vi "Agilent 364xA (GPIB,Serial) Initialization VI.vi"(8 "error in (no error)":errorcluster, 10 "Custom XML":string, 11 "Device Item Ref in":T3 format="%.0x") -> (0 "error out":errorcluster, 3 "Device Item Ref out":T3 format="%.0x")   [LabVIEW 2009, in "Agilent 364xA (GPIB,Serial) Custom Device.lvlib"]
uses:
  Agilent 364xA (GPIB,Serial) Custom Device.lvlib
  <vilib>/NI VeriStand/Custom Device API/Custom Device Item Ref.ctl
  <vilib>/NI VeriStand/Custom Device API/Custom Device Channel.ctl
  <vilib>/NI VeriStand/Custom Device API/Custom Device Channel Type.ctl
  <vilib>/NI VeriStand/Custom Device API/Custom Device Loop Type.ctl
  <vilib>/NI VeriStand/Custom Device API/Custom Device API.lvlib
panel:
  in  "Enable Channel":T1={"Type"=enum."Input", "Units"="", "Default Value"=0.0, "Faultable"=TRUE, "Scalable"=FALSE}
  in  "Output Channels":T1={"Type"=enum."Output", "Units"="", "Default Value"=0.0, "Faultable"=FALSE, "Scalable"=FALSE}
  in  "Input Channels":T1={"Type"=enum."Input", "Units"="Amps", "Default Value"=0.0, "Faultable"=TRUE, "Scalable"=TRUE}
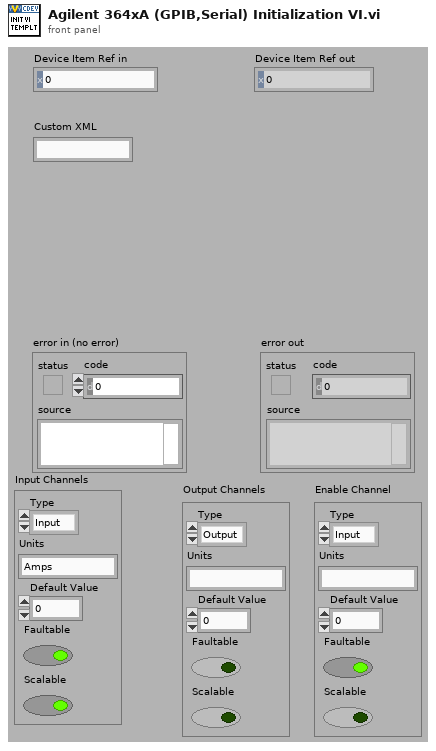
[diagram p1: front panel]
types:
  T1 = typedef "Custom Device API.lvlib/Custom Device Channel.ctl" = cluster{"Type":T2, "Units":string, "Default Value":dbl, "Faultable":bool, "Scalable":bool}
  T2 = typedef "Custom Device API.lvlib/Custom Device Channel Type.ctl" = enum16{"Input", "Output"}
  T3 = typedef "Custom Device API.lvlib/Custom Device Item Ref.ctl" = u64
  T4 = typedef "Custom Device API.lvlib/Custom Device Loop Type.ctl" = enum32{"While Loop", "Timed Loop"}
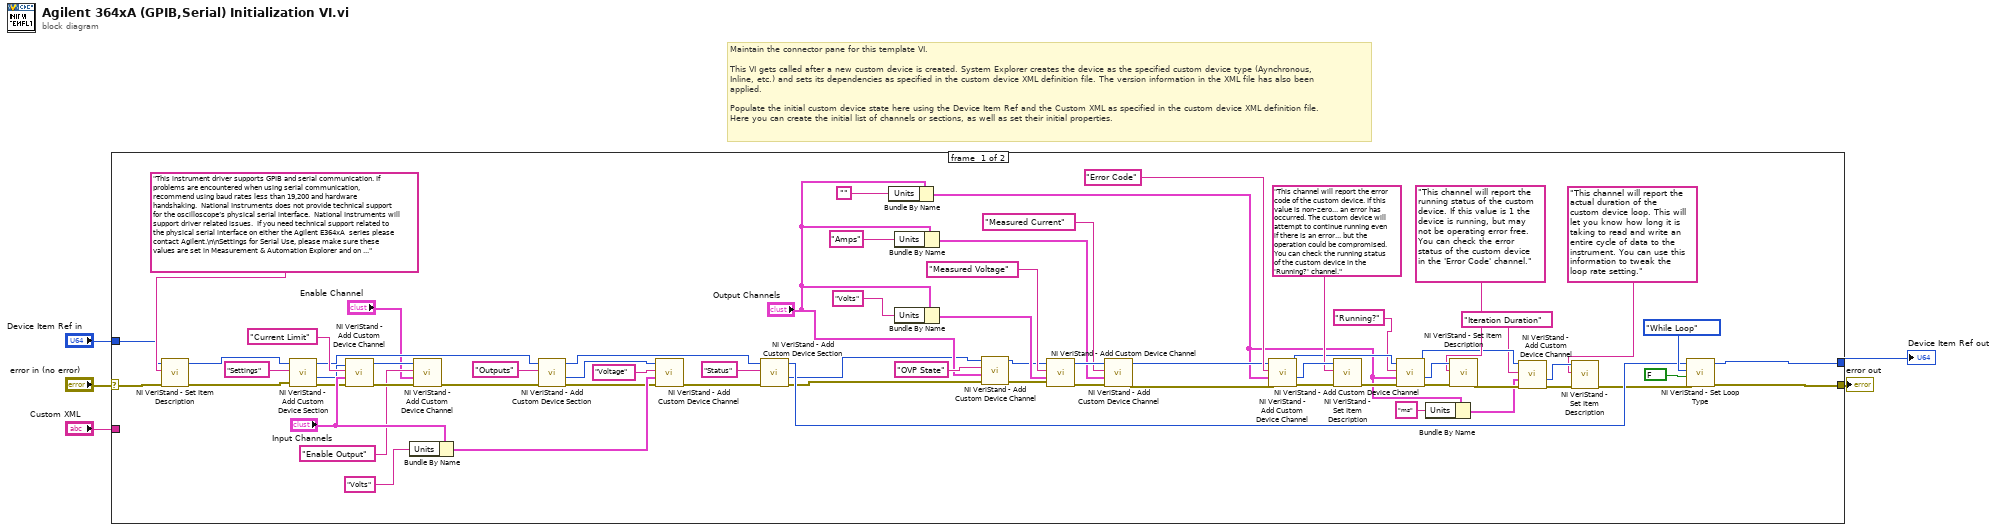
[diagram p0: block diagram]
diagram:
  # "Maintain the connector pane for this template VI.\n\nThis VI gets called after a new custom device is created. System Explorer creates the device as the specified custom device type (Aynchronous, Inline, etc.) and sets its dependencies as specified in the custom device XML definition file. The version information in the XML file has also been applied.\n\nPopulate the initial custom device state here using the Device Item Ref and the Custom XML as specified in the custom device XML definition file. Here you can create the initial list of channels or sections, as well as set their initial properties."
  n1 = case shown="No Error" "error in (no error)" {
    selector: "error in (no error)" -> [w30 w74]
    tunnel: [w7 w74] -> w5
    tunnel: [w6 w73] -> w3
    tunnel: "Device Item Ref in" -> [w27 w73]
    tunnel: "Custom XML" -> [_ _]
    frame #0 {
      n2 = call <vilib>:"NI VeriStand - Set Item Description.vi"("error in (no error)"=w30, "Description"="This instrument driver supports GPIB and serial communication. If problems are encountered when using serial communication, recommend using baud rates less than 19,200 and hardware handshaking.  National Instruments does not provide technical support for the oscilloscope’s physical serial interface.  National Instruments will support driver related issues.  If you need technical support related to the physical serial interface on either the Agilent E364xA  series please contact Agilent.\n\nSettings for Serial Use, please make sure these values are set in Measurement & Automation Explorer and on the instrument. Also be sure they match exactly with each other.\n\n-Baud Rate: 300, 600, 1200, 2400, 4800, or 9600 (factory setting) \n-Parity and Data Bit :  None / 8 data bits (factory setting), Even / 7 data bit , or Odd / 7 data bit \n-Number of  Start Bit : 1 bit (fixed on instrument) \n-Number of  Stop Bit :  2 bits (fixed on instrument) \n-Handshaking: DTR / DSR (fixed on instrument) ", "Item Ref in"=w27) -> ("error out"=w29:errorcluster, "Item Ref out"=w26:T3)  [unwired: 6 in, 1 out]
      n3 = call <vilib>:"NI VeriStand - Add Custom Device Section.vi"("error in (no error)"=w29, "Section Name"="Settings", "Parent Ref in"=w26) -> ("error out"=w51:errorcluster, "Section Ptr"=w54:T3, "Parent Ref out"=w47:T3)  [unwired: 6 in]
      n4 = call <vilib>:"NI VeriStand - Add Custom Device Channel.vi"("error in (no error)"=w51, "Channel"="Input Channels", "Channel Name"="Current Limit", "Parent Ref in"=w54) -> ("error out"=w48:errorcluster, "Parent Ref out"=w46:T3)  [unwired: 5 in, 1 out]
      n5 = Bundle By Name(cluster="Input Channels", "Units"="Volts") -> (w64:T1)
      n6 = call <vilib>:"NI VeriStand - Add Custom Device Channel.vi"("error in (no error)"=w48, "Channel"="Enable Channel", "Channel Name"="Enable Output", "Parent Ref in"=w46) -> ("error out"=w49:errorcluster)  [unwired: 5 in, 2 out]
      n7 = call <vilib>:"NI VeriStand - Add Custom Device Section.vi"("error in (no error)"=w49, "Section Name"="Outputs", "Parent Ref in"=w47) -> ("error out"=w50:errorcluster, "Section Ptr"=w53:T3, "Parent Ref out"=w68:T3)  [unwired: 6 in]
      n8 = call <vilib>:"NI VeriStand - Add Custom Device Channel.vi"("error in (no error)"=w50, "Channel"=w64, "Channel Name"="Voltage", "Parent Ref in"=w53) -> ("error out"=w69:errorcluster)  [unwired: 5 in, 2 out]
      n9 = call <vilib>:"NI VeriStand - Add Custom Device Section.vi"("error in (no error)"=w69, "Section Name"="Status", "Parent Ref in"=w68) -> ("error out"=w21:errorcluster, "Section Ptr"=w20:T3, "Parent Ref out"=w38:T3)  [unwired: 6 in]
      n10 = Bundle By Name(cluster="Output Channels", "Units"="") -> (w11:T1)
      n11 = Bundle By Name(cluster="Output Channels", "Units"="Amps") -> (w37:T1)
      n12 = Bundle By Name(cluster="Output Channels", "Units"="Volts") -> (w58:T1)
      n13 = call <vilib>:"NI VeriStand - Add Custom Device Channel.vi"("error in (no error)"=w21, "Channel"="Output Channels", "Channel Name"="OVP State", "Parent Ref in"=w20) -> ("error out"=w25:errorcluster, "Parent Ref out"=w24:T3)  [unwired: 5 in, 1 out]
      n14 = call <vilib>:"NI VeriStand - Add Custom Device Channel.vi"("error in (no error)"=w25, "Channel"=w58, "Channel Name"="Measured Voltage", "Parent Ref in"=w24) -> ("error out"=w61:errorcluster, "Parent Ref out"=w62:T3)  [unwired: 5 in, 1 out]
      n15 = call <vilib>:"NI VeriStand - Add Custom Device Channel.vi"("error in (no error)"=w61, "Channel"=w37, "Channel Name"="Measured Current", "Parent Ref in"=w62) -> ("error out"=w19:errorcluster, "Parent Ref out"=w18:T3)  [unwired: 5 in, 1 out]
      n16 = call <vilib>:"NI VeriStand - Add Custom Device Channel.vi"("error in (no error)"=w19, "Channel"=w11, "Channel Name"="Error Code", "Parent Ref in"=w18) -> ("error out"=w41:errorcluster, "Channel Ref"=w40:T3, "Parent Ref out"=w35:T3)  [unwired: 5 in]
      n17 = call <vilib>:"NI VeriStand - Set Item Description.vi"("error in (no error)"=w41, "Description"="This channel will report the error code of the custom device. If this value is non-zero... an error has occurred. The custom device will attempt to continue running even if there is an error... but the operation could be compromised. You can check the running status of the custom device in the 'Running?' channel.", "Item Ref in"=w40) -> ("error out"=w36:errorcluster)  [unwired: 6 in, 2 out]
      n18 = call <vilib>:"NI VeriStand - Add Custom Device Channel.vi"("error in (no error)"=w36, "Channel"=w11, "Channel Name"="Running?", "Parent Ref in"=w35) -> ("error out"=w34:errorcluster, "Channel Ref"=w33:T3, "Parent Ref out"=w15:T3)  [unwired: 5 in]
      n19 = Bundle By Name(cluster=w11, "Units"="ms") -> (w9:T1)
      n20 = call <vilib>:"NI VeriStand - Set Item Description.vi"("error in (no error)"=w34, "Description"="This channel will report the running status of the custom device. If this value is 1 the device is running, but may not be operating error free.  You can check the error status of the custom device in the 'Error Code' channel.", "Item Ref in"=w33) -> ("error out"=w16:errorcluster)  [unwired: 6 in, 2 out]
      n21 = call <vilib>:"NI VeriStand - Add Custom Device Channel.vi"("error in (no error)"=w16, "Channel"=w9, "Channel Name"="Iteration Duration", "Parent Ref in"=w15) -> ("error out"=w17:errorcluster, "Channel Ref"=w14:T3)  [unwired: 5 in, 1 out]
      n22 = call <vilib>:"NI VeriStand - Set Item Description.vi"("error in (no error)"=w17, "Description"="This channel will report the actual duration of the custom device loop. This will let you know how long it is taking to read and write an entire cycle of data to the instrument. You can use this information to tweak the loop rate setting.", "Item Ref in"=w14) -> ("error out"=w13:errorcluster)  [unwired: 6 in, 2 out]
      n23 = call <vilib>:"NI VeriStand - Set Loop Type.vi"("error in (no error)"=w13, "Use Device Clock (Timed Loops only)"=FALSE, "Loop type"=Custom_Device_Loop_Type."While Loop", "Device Ref in"=w38) -> ("error out"=w7:errorcluster, "Device Ref out"=w6:T3)  [unwired: 6 in]
    }
    frame #1 {
    }
  }
  "error out" <- w5
  "Device Item Ref out" <- w3
